vi "FileCreate.vi"(8 "error in 2":errorcluster, 11 "DAQ File Name":string) -> (0 "error out 2":errorcluster, 3 "appended path 2":path)   [LabVIEW 2019, in "2231A.lvclass"]
uses:
  2231A.lvclass
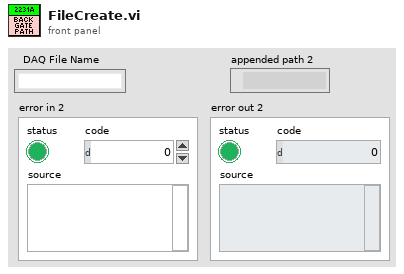
[diagram p1: front panel]
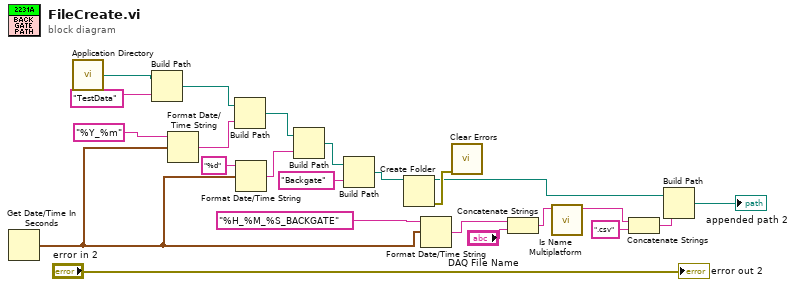
[diagram p0: block diagram]
diagram:
  n1 = Get Date/Time In Seconds() -> (seconds since 1Jan1904=w19:timestamp)
  n2 = call <vilib>:"Application Directory.vi"() -> ("Application Directory"=w8:path)
  n3 = Build Path(base path=w8, name or relative path="TestData") -> (appended path=w17:path)
  n4 = Format Date/Time String(time format string (%c)="%Y_%m", seconds (now)=w19) -> (date/time string=w16:string)  [unwired: 1 in]
  n5 = Build Path(base path=w17, name or relative path=w16) -> (appended path=w18:path)
  n6 = Format Date/Time String(time format string (%c)="%d", seconds (now)=w19) -> (date/time string=w4:string)  [unwired: 1 in]
  n7 = Build Path(base path=w18, name or relative path=w4) -> (appended path=w3:path)
  n8 = Build Path(base path=w3, name or relative path="Backgate") -> (appended path=w1:path)
  n9 = Create Folder(path (use dialog)=w1) -> (created path=w11:path, error out=w12:errorcluster)  [unwired: 2 in, 1 out]
  n10 = Format Date/Time String(time format string (%c)="%H_%M_%S_BACKGATE", seconds (now)=w19) -> (date/time string=w6:string)  [unwired: 1 in]
  n11 = call <vilib>:"Clear Errors.vi"("error in (no error)"=w12) -> ()  [unwired: 5 in, 2 out]
  n12 = Concatenate Strings(w6, "DAQ File Name") -> (w10:string)
  n13 = call <vilib>:"Is Name Multiplatform.vi"("filename"=w10) -> ("suggested filename"=w22:string)  [unwired: 6 in, 4 out]
  n14 = Concatenate Strings(w22, ".csv" ("string")) -> (w23:string)
  n15 = Build Path(base path=w11, name or relative path=w23) -> (appended path=→"appended path 2":path)
  "error out 2" <- "error in 2"
